vi "Test Coffee Shop Add Barista Broadcast Name.vi"(8 "error in (no error)":errorcluster, 11 "Coffee Shop Test In":refnum<class "Coffee Shop Test.lvclass">) -> (0 "error out":errorcluster, 3 "Coffee Shop Test Out":refnum<class "Coffee Shop Test.lvclass">)   [LabVIEW 2020, in "Coffee Shop Test.lvclass"]
uses:
  Coffee Shop Test.lvclass
  Coffee Shop/Coffee Shop.lvclass
  <vilib>/Asteme/Triarc Framework/Process/Process.lvclass
  C:/Program Files (x86)/National Instruments/LabVIEW 2020/vi.lib/Asteme/Triarc Framework/Application/Application.lvclass
  C:/Program Files (x86)/National Instruments/LabVIEW 2020/vi.lib/Asteme/Triarc Framework/Process/Process.lvclass
  C:/Program Files (x86)/National Instruments/LabVIEW 2020/vi.lib/Asteme/Triarc Framework/Base/Base.lvclass
  C:/Program Files (x86)/National Instruments/LabVIEW 2020/vi.lib/Asteme/Triarc Framework/Error Handler Interface/Error Handler Interface.lvclass
  C:/Program Files (x86)/National Instruments/LabVIEW 2020/vi.lib/Asteme/Triarc Framework/Logging/Logging.lvclass
  C:/Users/anton/Documents/GitHub/Triarc-Examples/Coffee Shop/Coffee Shop/Coffee Shop.lvclass
  <vilib>/Asteme/Triarc Framework Test Suite/Support/Event Helpers/Event Helpers.lvlib
  <vilib>/Asteme/LUnit/Test Case.lvclass
  C:/Program Files (x86)/National Instruments/LabVIEW 2020/vi.lib/Asteme/Triarc Framework Test Suite/Application Test/Application Test.lvclass
  C:/Program Files (x86)/National Instruments/LabVIEW 2020/vi.lib/Asteme/Triarc Framework Test Suite/Process Test/Process Test.lvclass
  C:/Program Files (x86)/National Instruments/LabVIEW 2020/vi.lib/Asteme/Triarc Framework Test Suite/Base Class Test/Base Test.lvclass
  C:/Program Files (x86)/National Instruments/LabVIEW 2020/vi.lib/Asteme/LUnit/Test Case.lvclass
  C:/Users/anton/Documents/GitHub/Triarc-Examples/Coffee Shop/Coffee Shop Test/Coffee Shop Test.lvclass
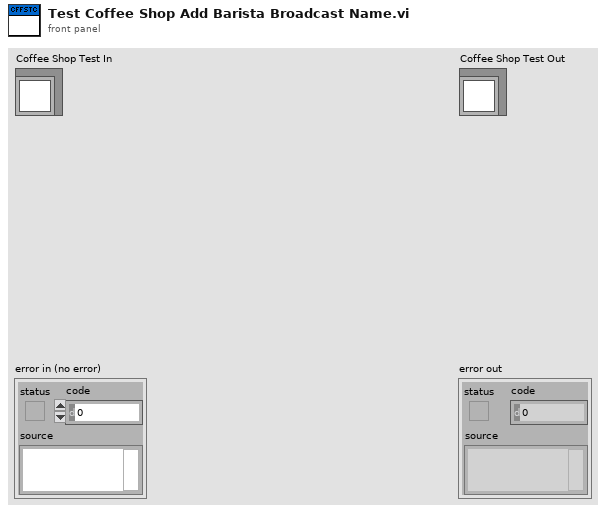
[diagram p1: front panel]
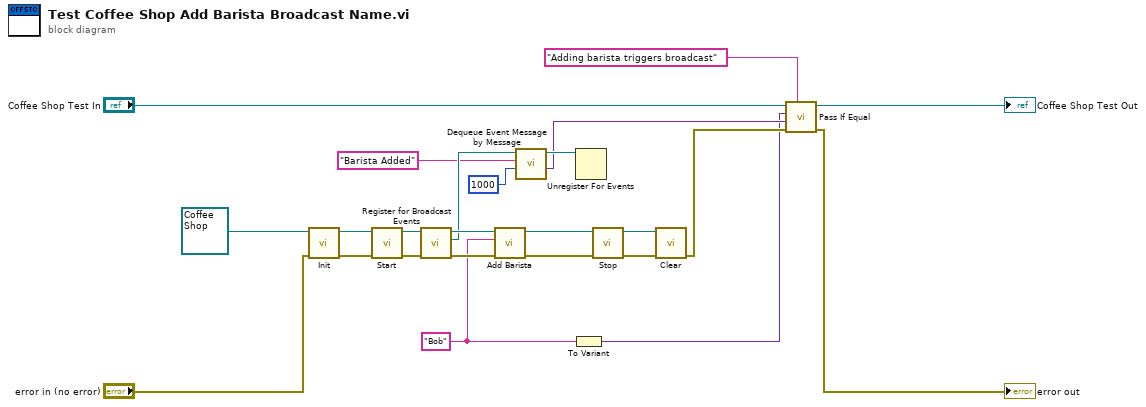
[diagram p0: block diagram]
diagram:
  w2 = "Bob" ("Name")
  n1 = call-dynamic "Init.vi"("error in (no error)"="error in (no error)", "Process In"=refnum<class "Coffee Shop.lvclass"> refnum ("Coffee Shop.lvclass")) -> ("error out"=w22:errorcluster, "Process Out"=w23:refnum<class "Coffee Shop.lvclass">)  [unwired: 8 in]
  n2 = call <vilib>:"Start.vi"("error in (no error)"=w22, "Process In"=w23) -> ("error out"=w21:errorcluster, "Process Out"=w14:refnum<class "Coffee Shop.lvclass">)  [unwired: 8 in]
  n3 = call <vilib>:"Register for Broadcast Events.vi"("error in (no error)"=w21, "Process In"=w14) -> ("error out"=w15:errorcluster, "Event Registration Refnum Out"=w12:refnum<event-registration>, "Process Out"=w13:refnum<class "Coffee Shop.lvclass">)  [unwired: 7 in]
  n4 = call "Add Barista.vi"("error in (no error)"=w15, "Name"=w2, "Coffee Shop in"=w13) -> ("error out"=w17:errorcluster, "Coffee Shop out"=w16:refnum<class "Coffee Shop.lvclass">)  [unwired: 7 in]
  n5 = call <vilib>:"Dequeue Event Message by Message.vi"("Timeout (-1)"=1000, "Message"="Barista Added", "Event Registration Refnum"=w12) -> ("Message Data"=w3:variant, "Event Registration Refnum Out"=w10:refnum<event-registration>)  [unwired: 4 in, 3 out]
  n6 = To Variant(anything=w2) -> (Variant=w1:variant)
  n7 = Unregister For Events(event registration refnum=w10) -> ()  [unwired: 1 in, 1 out]
  n8 = call <vilib>:"Stop.vi"("error in (no error)"=w17, "Process In"=w16) -> ("error out"=w19:errorcluster, "Process Out"=w20:refnum<class "Coffee Shop.lvclass">)  [unwired: 7 in, 1 out]
  n9 = call-dynamic "Clear.vi"("error in (no error)"=w19, "Application In"=w20) -> ("error out"=w6:errorcluster)  [unwired: 9 in]
  n10 = call <vilib>:"Pass If Equal.vi"("Description"="Adding barista triggers broadcast", "error in (no error)"=w6, "Actual"=w3, "Expected"=w1, "Test Case In"="Coffee Shop Test In") -> ("error out"=→"error out":errorcluster, "Test Case Out"=→"Coffee Shop Test Out":refnum<class "Coffee Shop Test.lvclass">)  [unwired: 5 in]
